vi "SCT CBD CheckIfExists.vi"(10 "Items To Add":string[](array[string]) caption="添加项", 11 "Existing Items":string[](array[string]) caption="现有项") -> (3 "Exists?":bool caption="存在？")   [LabVIEW 2016]
panel:
  in  "message":string="无法创建绑定变量。名称必须以Custom为基，且不能\n与上级库中的项重名。\n" caption="消息"
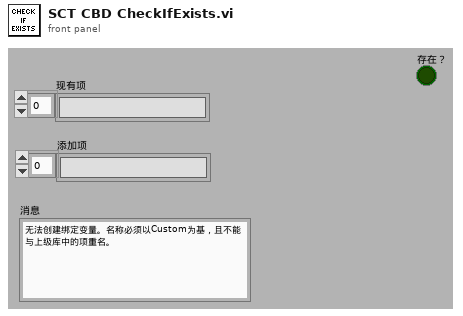
[diagram p1: front panel]
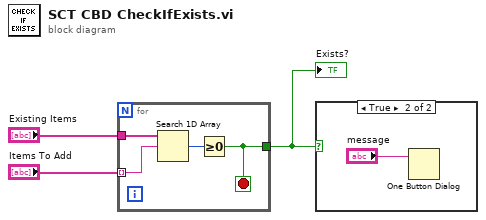
[diagram p0: block diagram]
diagram:
  n1 = for {
    tunnel: "Items To Add" -> [w5] mode=indexing
    tunnel: "Existing Items" -> [w7]
    tunnel: [w4] -> w1
    stop <- w4 stop-if-true
    n2 = Search 1D Array(1D array=w7, element=w5) -> (index of element=w6:i32)  [unwired: 1 in]
    n3 = Greater Or Equal To 0?(x=w6) -> (x >= 0?=w4:bool)
  }
  "Exists?" <- w1
  n4 = case shown="True" w1 {
    frame False {
    }
    frame True {
      n5 = One Button Dialog(message="message") -> ()  [unwired: 1 in, 1 out]
    }
  }
